vi "test10-StateChange_Event.vi"(8 "error in (no error)":errorcluster, 11 "TestCase in":refnum<class "testcase-CSMGlobalLog.lvclass">) -> (0 "error out":errorcluster, 3 "TestCase out":refnum<class "testcase-CSMGlobalLog.lvclass">)   [LabVIEW 2017, in "testcase-CSMGlobalLog.lvclass"]
uses:
  testcase-CSMGlobalLog.lvclass
  testcase-CSMGlobalLog.lvclass/testcase-CSMGlobalLog.ctl
  src/user.lib/_NEVSTOP/Communicable State Machine(CSM)/_Support/Typedef/_CSM_GlobalLog_MSG.ctl
  src/user.lib/_NEVSTOP/Communicable State Machine(CSM)/_Support/Typedef/_CSM_Response Source Message.ctl
  src/user.lib/_NEVSTOP/Communicable State Machine(CSM)/_Support/Typedef/_CSM_GlobalLog_MSG_TYPE.ctl
  24a778c7-405f-47d7-a6be-afdb60495ae4.vi
  src/user.lib/_NEVSTOP/Communicable State Machine(CSM)/_Support/GlobalEvent/GEvt-Generate with Rule Check.vi
  src/user.lib/_NEVSTOP/Communicable State Machine(CSM)/AdvanceAPI/CSM - Convert Error to Argument.vi
  src/user.lib/_NEVSTOP/Communicable State Machine(CSM)/AdvanceAPI/CSM - Make String Arguments Safe.vi
  src/user.lib/_NEVSTOP/Communicable State Machine(CSM)/AdvanceAPI/CSM - Keywords.vi
  src/user.lib/_NEVSTOP/Communicable State Machine(CSM)/_Support/GlobalEvent/Cache-GEvt Refs.vi
  src/user.lib/_NEVSTOP/Communicable State Machine(CSM)/_Support/GlobalEvent/LogFilter/LogFilter - Check.vi
  src/user.lib/_NEVSTOP/Communicable State Machine(CSM)/_Support/GlobalEvent/LogFilter/LogFilter.lvclass
  <vilib>/addons/_JKI Toolkits/VI Tester/TestCase.llb/TestCase.lvclass
  src/user.lib/_NEVSTOP/Communicable State Machine(CSM)/Communicable State Machine.lvlib
  CSM/CSM-Testcase.lvlib
  C:/Program Files (x86)/National Instruments/LabVIEW 2017/vi.lib/addons/_JKI Toolkits/VI Tester/TestCase.llb/TestCase.lvclass
panel:
  out "String Cache Each Loop":string
  out "LoopCount":i32
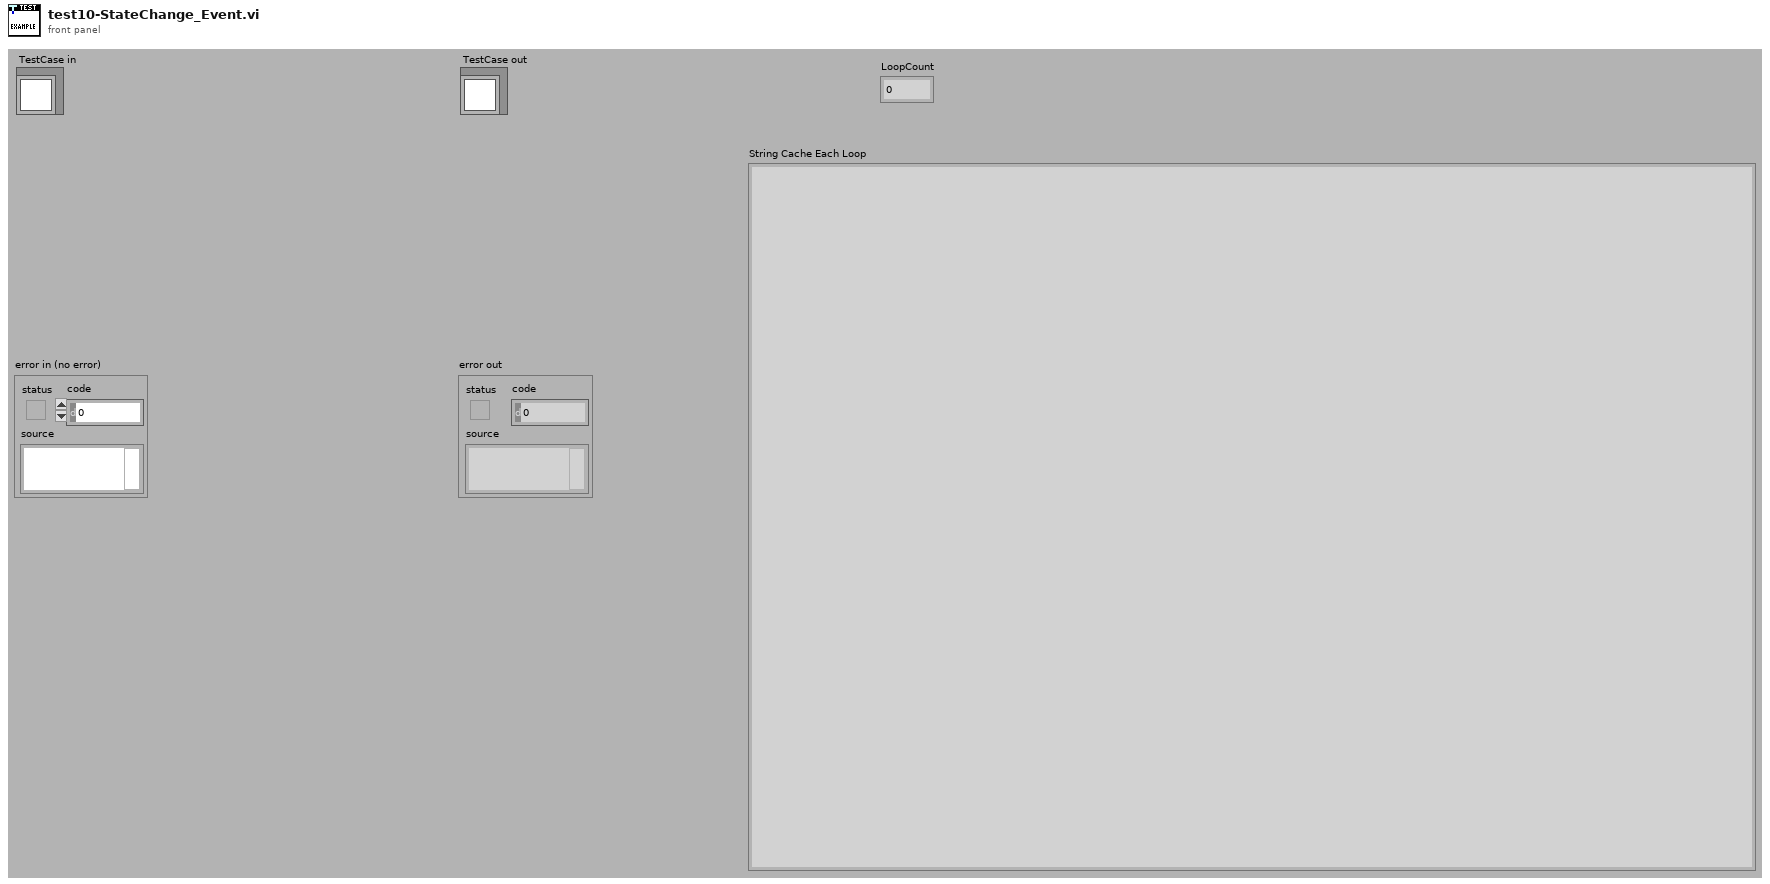
[diagram p1: front panel]
types:
  T1 = typedef "Communicable State Machine.lvlib/_CSM_GlobalLog_MSG.ctl" = cluster{"Name (\"\" to Use UUID)":string, "Current State":string, "Arguments":string, "Source Message":T2, "Source Module":string, "Complete(T)/Start(F)":bool, "LogType":T3, "Time Stamp":timestamp}
  T2 = typedef "Communicable State Machine.lvlib/_CSM_Response Source Message.ctl" = cluster{"‘State":string, "’Arguments":string, "’Error":errorcluster}
  T3 = typedef "Communicable State Machine.lvlib/_CSM_GlobalLog_MSG_TYPE.ctl" = enum16{"User Log", "State Change", "Status", "Interrupt", "Register", "Unregister", "Error Log", "Module Created", "Module Destroyed", "Async Message", "No-Rep Async Message", "Sync Message"}
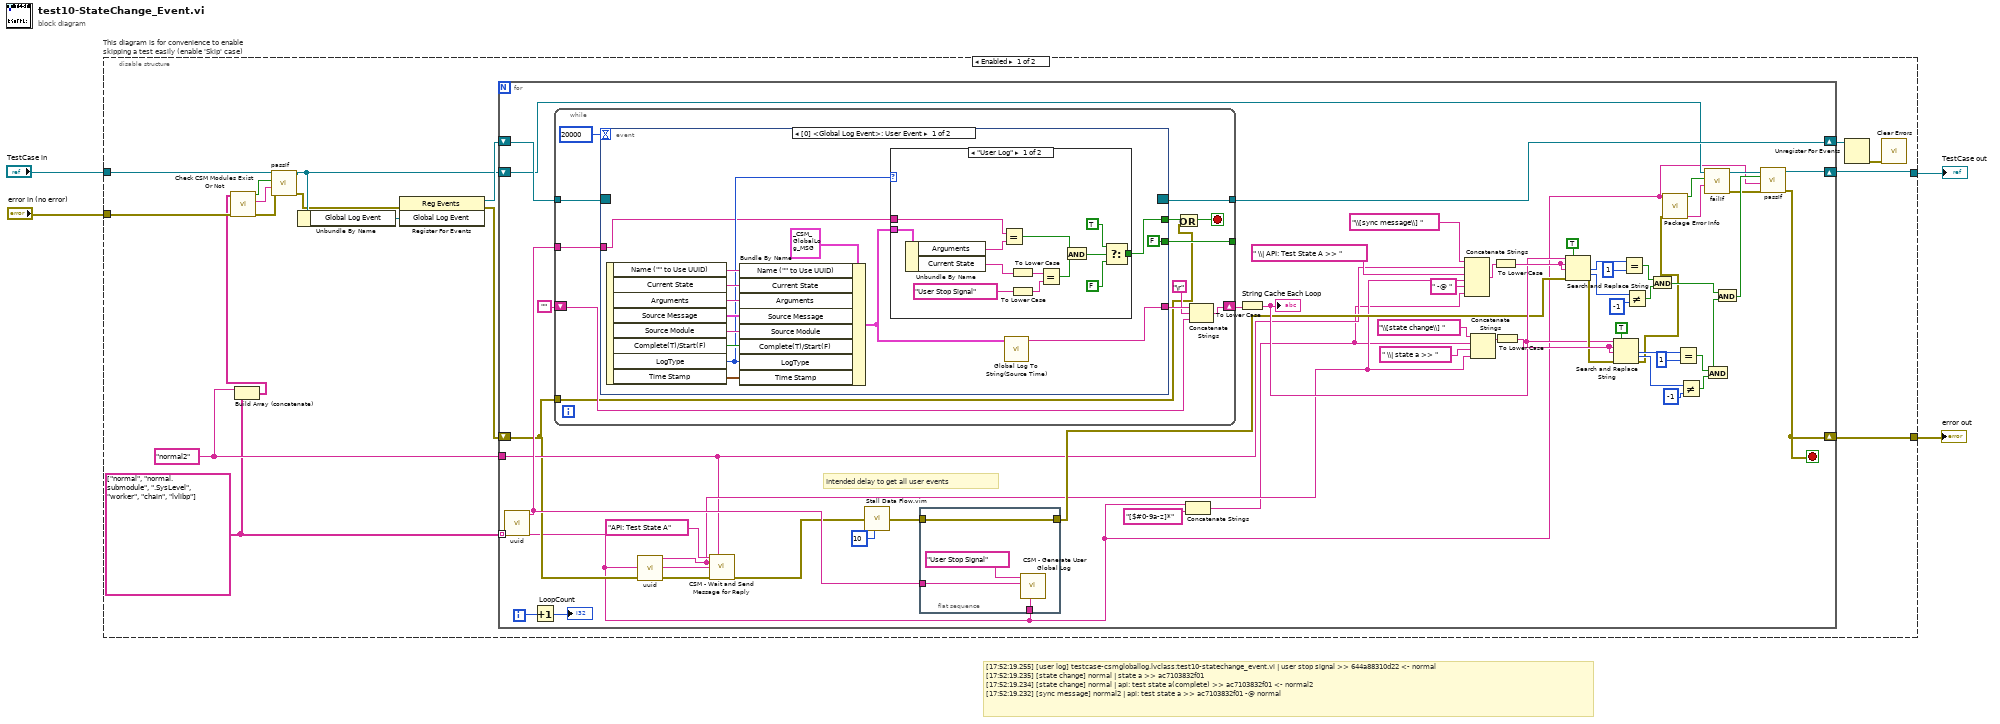
[diagram p0: block diagram]
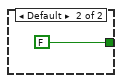
[diagram p2: hidden frame]
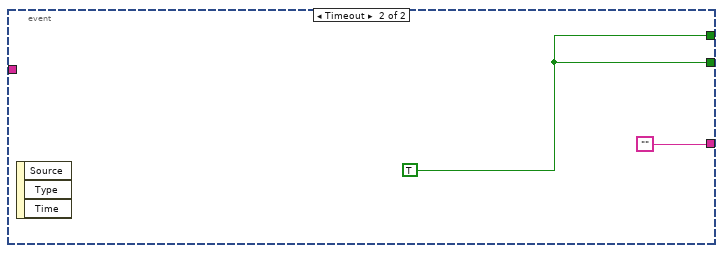
[diagram p3: hidden frame]
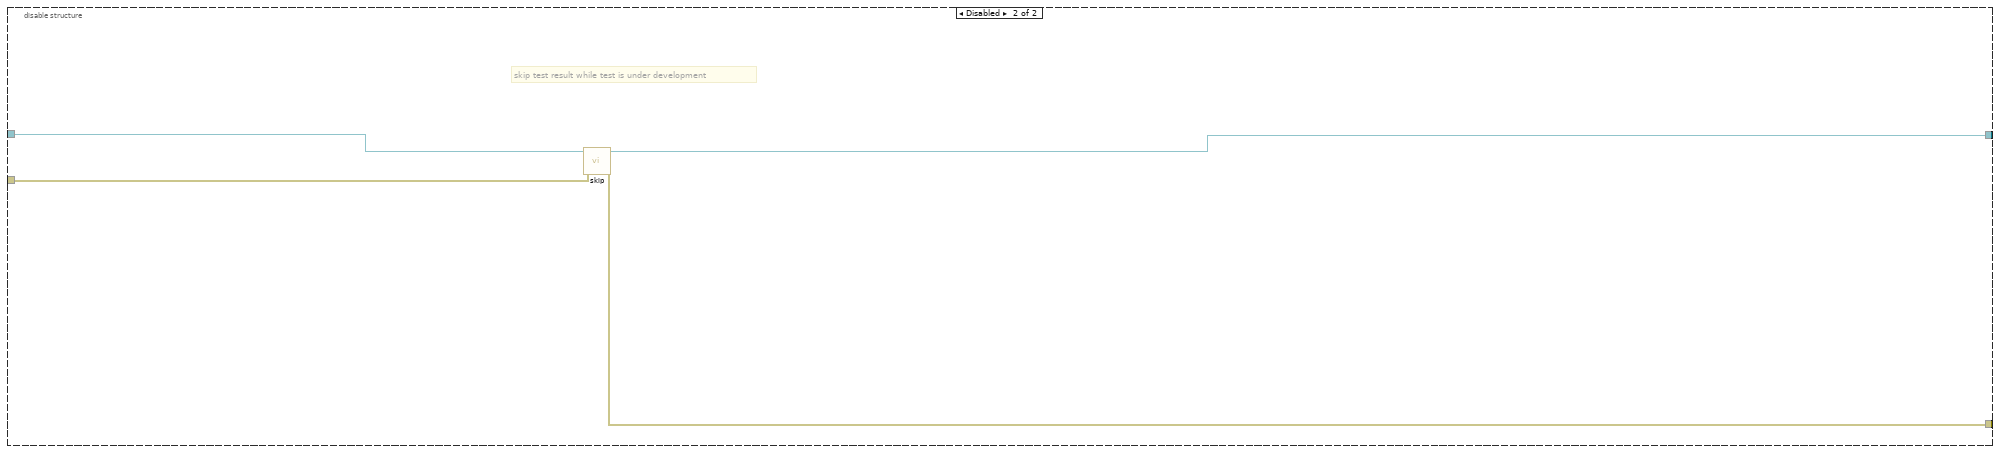
[diagram p4: hidden frame]
diagram:
  # "[17:52:19.255] [user log] testcase-csmgloballog.lvclass:test10-statechange_event.vi | user stop signal >> 644a88310d22 <- normal\n[17:52:19.235] [state change] normal | state a >> ac7103832f01\n[17:52:19.234] [state change] normal | api: test state a(complete) >> ac7103832f01 <- normal2\n[17:52:19.232] [sync message] normal2 | api: test state a >> ac7103832f01 -@ normal"
  n1 = disable-structure "This diagram is for convenience to enable skipping a test easily (enable 'Skip' case)" shown="Enabled" {
    disable-tunnel: "TestCase in" -> [w13 w125]
    disable-tunnel: [w17 w123] -> w1
    disable-tunnel: [w16 w124] -> w3
    disable-tunnel: "error in (no error)" -> [w11 w122]
    frame Enabled {
      w10 = "normal2" ("CSM")
      w9 = string[] ["normal", "normal.submodule", ".SysLevel", "worker", "chain", "lvlibp"]
      n2 = Build Array (concatenate)(w10, w9) -> (w8:string[])
      n3 = call "Check CSM Modules Exist Or Not.vi"("error in"=w11, "CSM names in"=w8) -> ("error out"=w7:errorcluster, "Debug string"=w14:string, "All Modules Exist?"=w15:bool)  [unwired: 7 in]
      n4 = call-dynamic "passIf.vi"("error in (no error)"=w7, "message (\"\")"=w14, "pass"=w15, "TestCase in"=w13) -> ("error out"=w6:errorcluster, "TestCase out"=w12:refnum<class "testcase-CSMGlobalLog.lvclass">)  [unwired: 6 in]
      n5 = Unbundle By Name(w12) -> ("Global Log Event"=w21:refnum<user-event>)
      n6 = register-events(error in=w6, w21) -> (reference out=w20:refnum<event-registration>, error out=w18:errorcluster)  [unwired: 1 in]
      n7 = for {
        shift-right: [w74] -> w19
        shift-left: w20 -> [w75]
        shift-right: [w70] -> w16
        shift-left: w18 -> [w29]
        tunnel: w9 -> [w22] mode=indexing
        shift-right: [w73] -> w17
        shift-left: w12 -> [w23]
        tunnel: w10 -> [w31]
        i -> [w72]
        stop <- w70 stop-if-true
        # "Intended delay to get all user events"
        n8 = call "uuid.vi"() -> ("UUID"=w69:string)  [unwired: 11 in]
        n9 = Increment(x=w72) -> (x+1=→"LoopCount":i32)
        n10 = while {
          tunnel: w75 -> [w91]
          tunnel: [w90] -> w74
          shift-right: [w84] -> w66
          shift-left: "" -> [w86]
          tunnel: w69 -> [w88]
          tunnel: [w87] -> _
          tunnel: w29 -> [w80]
          stop <- w82 stop-if-true
          n11 = event shown="[0] <Global Log Event>: User Event" {
            selector: w91 -> [_ _]
            dyn-events: [_ _] -> w90
            timeout: 20000 -> [_ _]
            tunnel: [w92 ""] -> w85
            tunnel: [w94 w121] -> w81
            tunnel: w88 -> [w95 _]
            tunnel: [FALSE ("Stop") w121] -> w87
            event User Event {
              n12 = event-data() -> ("Name (\"\" to Use UUID)"=w104:string, "Current State"=w103:string, "Arguments"=w102:string, "Source Message"=w101:T2, "Source Module"=w100:string, "Complete(T)/Start(F)"=w99:bool, "LogType"=w96:T3, "Time Stamp"=w98:timestamp)  [unwired: 1 in]
              n13 = Bundle By Name(cluster=T1 {"Name (\"\" to Use UUID)"="", "Current State"="", "Arguments"="", "Source Message"={"‘State"="", "’Arguments"="", "’Error"={"status"=FALSE, "code"=0, "source"=""}}, "Source Module"="", "Complete(T)/Start(F)"=FALSE, "LogType"=enum."State Change", "Time Stamp"=timestamp(0 s since 1904-01-01)} ("Cross CSM Data"), "Name (\"\" to Use UUID)"=w104, "Current State"=w103, "Arguments"=w102, "Source Message"=w101, "Source Module"=w100, "Complete(T)/Start(F)"=w99, "LogType"=w96, "Time Stamp"=w98) -> (w93:T1)
              n14 = case shown="\"User Log\"" w96 {
                tunnel: w93 -> [w118 _]
                tunnel: w95 -> [w117 _]
                tunnel: [w106 FALSE] -> w94
                frame "User Log" {
                  n15 = Unbundle By Name(w118) -> ("Arguments"=w116:string, "Current State"=w115:string)
                  n16 = Equal?(x=w117, y=w116) -> (x = y?=w110:bool)
                  n17 = To Lower Case(string=w115) -> (all lower case string=w114:string)
                  n18 = To Lower Case(string="User Stop Signal" ("Log")) -> (all lower case string=w112:string)
                  n19 = Equal?(x=w114, y=w112) -> (x = y?=w111:bool)
                  n20 = And(x=w110, y=w111) -> (x .and. y?=w109:bool)
                  n21 = Select(t=TRUE, s=w109, f=FALSE) -> (s? t:f=w106:bool)
                }
                frame Default {
                }
              }
              n22 = call "Global Log To String(Source Time).vi"("Log"=w93) -> ("Log String"=w92:string)  [unwired: 9 in]
            }
            event Timeout {
              w121 = TRUE ("Stop")
              n23 = event-data() -> ()  [unwired: 1 in, 3 out]
            }
          }
          n24 = Or(x=w81, y=w80) -> (x .or. y?=w82:bool)
          n25 = Concatenate Strings(w85, "\r", w86) -> (w84:string)
        }
        n26 = call "uuid.vi"() -> ("UUID"=w35:string)  [unwired: 11 in]
        n27 = call "CSM - Wait and Send Message for Reply.vi"("State"="API: Test State A", "Current Module (\"\" to Generate an ID)"=w31, "Arguments (\"\")"=w35, "Target Module"=w22, "Error In (No Error)"=w29) -> ("error out"=w64:errorcluster)  [unwired: 7 in, 3 out]
        n28 = call "Stall Data Flow.vim"("value in"=w64, "milliseconds to wait"=u32 10) -> ("value out"=w67:errorcluster)  [unwired: 1 out]
        n29 = flat-sequence {
          tunnel: w67 -> [w76]
          tunnel: [w76] -> w36
          tunnel: w69 -> [w78]
          tunnel: w22 -> [w77]
          frame #0 {
            n30 = call "CSM - Generate User Global Log.vi"("From Who"=w77, "Arguments"=w78, "Log"="User Stop Signal") -> ()  [unwired: 8 in, 1 out]
          }
        }
        n31 = Concatenate Strings(w22, "[$#0-9a-z]*" ("string")) -> (w30:string)
        n32 = To Lower Case(string=w66) -> (all lower case string=w38:string)
        "String Cache Each Loop" <- w38
        n33 = Concatenate Strings("\\[sync message\\] " ("regular expression"), w31, " \\| API: Test State A >> " ("string"), w35, " -@ " ("string"), w30) -> (w60:string)
        n34 = Concatenate Strings("\\[state change\\] " ("regular expression"), w30, " \\| state a >> " ("string"), w35) -> (w62:string)
        n35 = To Lower Case(string=w60) -> (all lower case string=w58:string)
        n36 = To Lower Case(string=w62) -> (all lower case string=w47:string)
        n37 = Search and Replace String(replace all?=TRUE ("replace all? (F)"), input string=w38, search string=w58, replace string=w58, error in=w36) -> (number of replacements=w57:i32, offset past replacement=w56:i32, error out=w46:errorcluster)  [unwired: 3 in, 1 out]
        n38 = Search and Replace String(replace all?=TRUE ("replace all? (F)"), input string=w38, search string=w47, replace string=w47, error in=w46) -> (number of replacements=w49:i32, offset past replacement=w50:i32, error out=w26:errorcluster)  [unwired: 3 in, 1 out]
        n39 = Equal?(x=w57, y=1) -> (x = y?=w54:bool)
        n40 = Not Equal?(x=w56, y=-1) -> (x != y?=w53:bool)
        n41 = And(x=w54, y=w53) -> (x .and. y?=w40:bool)
        n42 = call "Package Error Info.vi"("error in"=w26, "String in"=w22) -> ("packed error info out"=w27:string, "error status"=w28:bool)  [unwired: 8 in]
        n43 = Equal?(x=w49, y=1) -> (x = y?=w51:bool)
        n44 = Not Equal?(x=w50, y=-1) -> (x != y?=w52:bool)
        n45 = call-dynamic "failIf.vi"("message (\"\")"=w27, "fail"=w28, "TestCase in"=w23) -> ("error out"=w25:errorcluster, "TestCase out"=w24:refnum<class "testcase-CSMGlobalLog.lvclass">)  [unwired: 7 in]
        n46 = And(x=w51, y=w52) -> (x .and. y?=w45:bool)
        n47 = And(x=w40, y=w45) -> (x .and. y?=w33:bool)
        n48 = call-dynamic "passIf.vi"("error in (no error)"=w25, "message (\"\")"=w22, "pass"=w33, "TestCase in"=w24) -> ("error out"=w70:errorcluster, "TestCase out"=w73:refnum<class "testcase-CSMGlobalLog.lvclass">)  [unwired: 6 in]
      }
      n49 = Unregister For Events(event registration refnum=w19) -> (error out=w5:errorcluster)  [unwired: 1 in]
      n50 = call <vilib>:"Clear Errors.vi"("error in (no error)"=w5) -> ()  [unwired: 5 in, 2 out]
    }
    frame Disabled {
      # "skip test result while test is under development"
      n51 = call <vilib>:"skip.vi"("error in (no error)"=w122, "TestCase in"=w125) -> ("error out"=w124:errorcluster, "TestCase out"=w123:refnum<class "testcase-CSMGlobalLog.lvclass">)  [unwired: 8 in]
    }
  }
  "error out" <- w3
  "TestCase out" <- w1
